vi "Power encode.vi"(11 "Array":dbl[](array[numeric])=[111.12345886230469, 111.12345886230469, 111.12345886230469, 9199.099609375, 9299.2001953125, 9399.5, 9499.599609375, 9599.7001953125, 9699.7998046875, 9799.900390625] format="%#.8g") -> (3 "Power string":string)   [LabVIEW 2021]
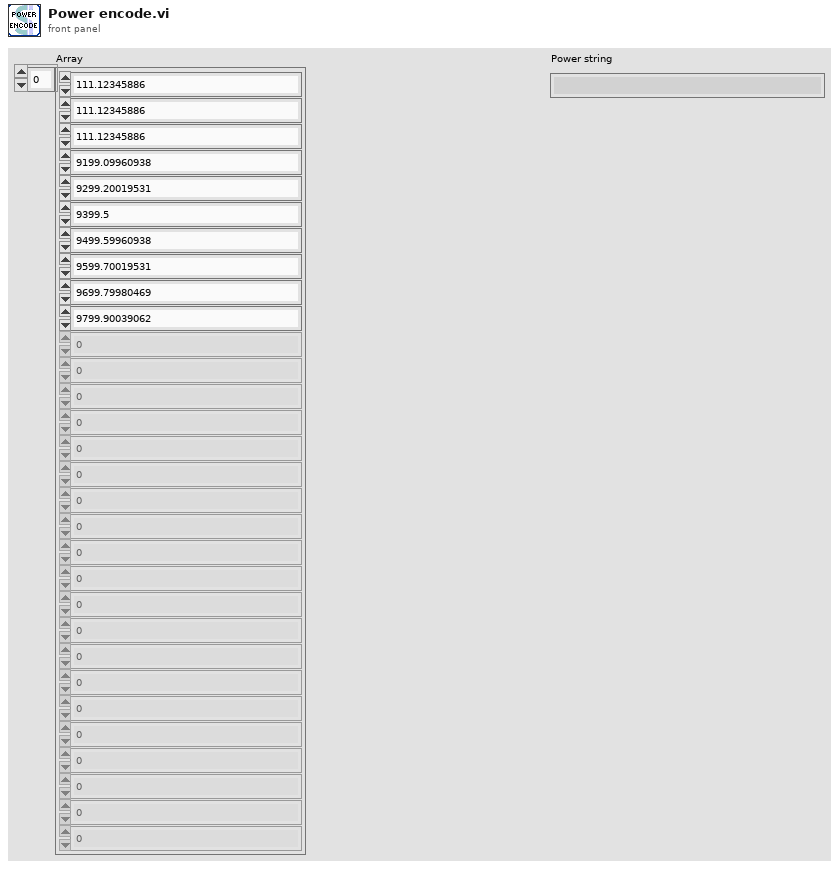
[diagram p1: front panel]
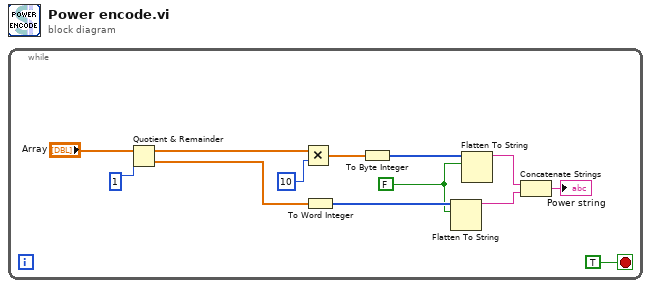
[diagram p0: block diagram]
diagram:
  n1 = while {
    stop <- TRUE stop-if-true
    w1 = FALSE ("prepend array or string size? (T)")
    n2 = Quotient & Remainder(x="Array", y=1) -> (x-y*floor(x/y)=w11:dbl[], floor(x/y)=w8:dbl[])
    n3 = Multiply(x=w11, y=10) -> (x*y=w9:dbl[])
    n4 = To Word Integer(number=w8) -> (16bit integer=w7:i16[])
    n5 = To Byte Integer(number=w9) -> (8bit integer=w6:i8[])
    n6 = Flatten To String(anything=w7, prepend array or string size? (T)=w1) -> (data string=w4:string)  [unwired: 2 in, 2 out]
    n7 = Flatten To String(anything=w6, prepend array or string size? (T)=w1) -> (data string=w5:string)  [unwired: 2 in, 2 out]
    n8 = Concatenate Strings(w5, w4) -> (→"Power string":string)
  }
